vi "Multiple_Windows.vi"() -> ()   [LabVIEW 2013]
uses:
  Global 2.vi
panel:
  in  "Input2":enum32{"Input2"}(tab)
  in  "OK Input 2":bool
  out "Input2_A":dbl
  out "Input2_B":dbl
  out "Input1":enum32{"Input1"}(tab)
  in  "OK Input 1":bool
  out "Input1_A":dbl
  out "Input1_B":dbl
  out "Input1 4":enum32{"Home"}(tab)
  in  "OK Input 3":bool
  in  "close":bool
  in  "Tab Control":enum32{"Home", "Input1", "Input2"}(tab)
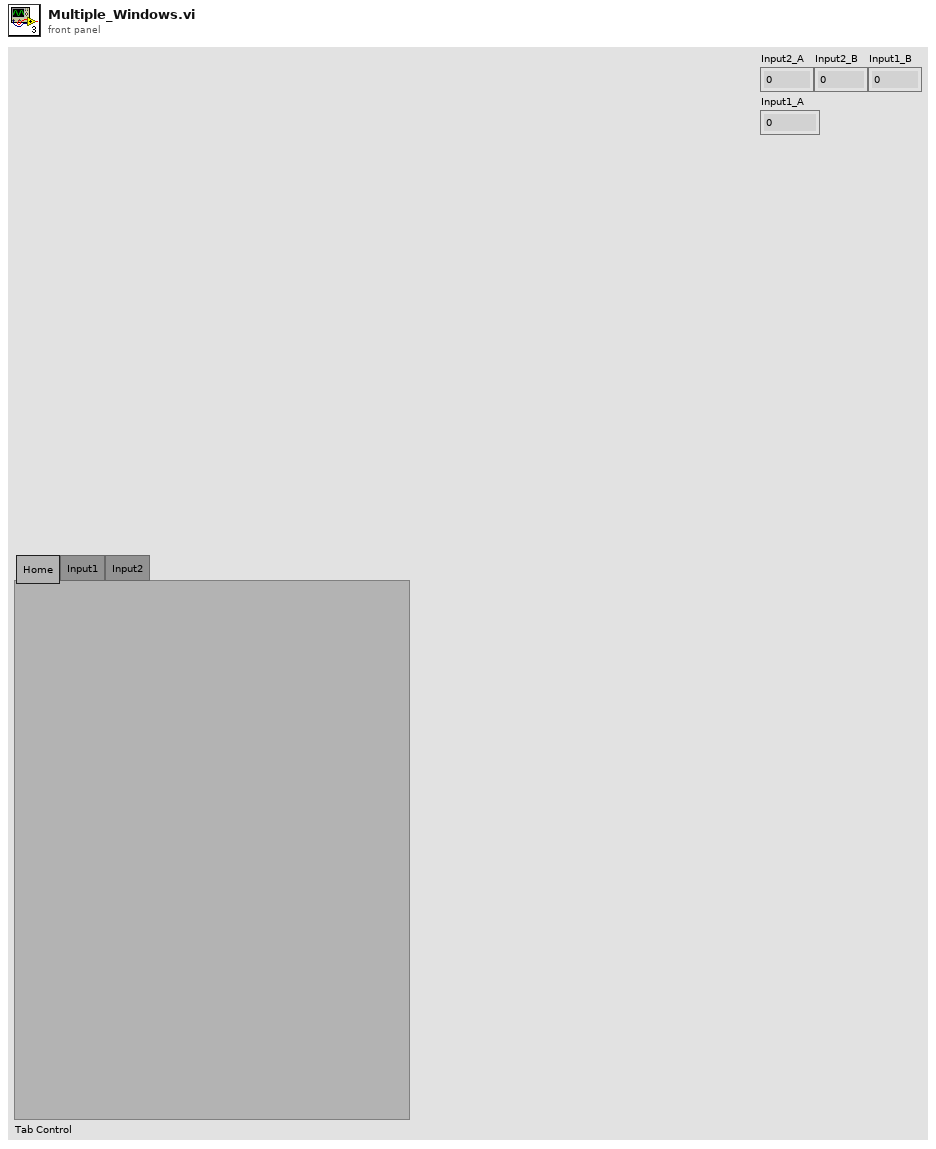
[diagram p1: front panel]
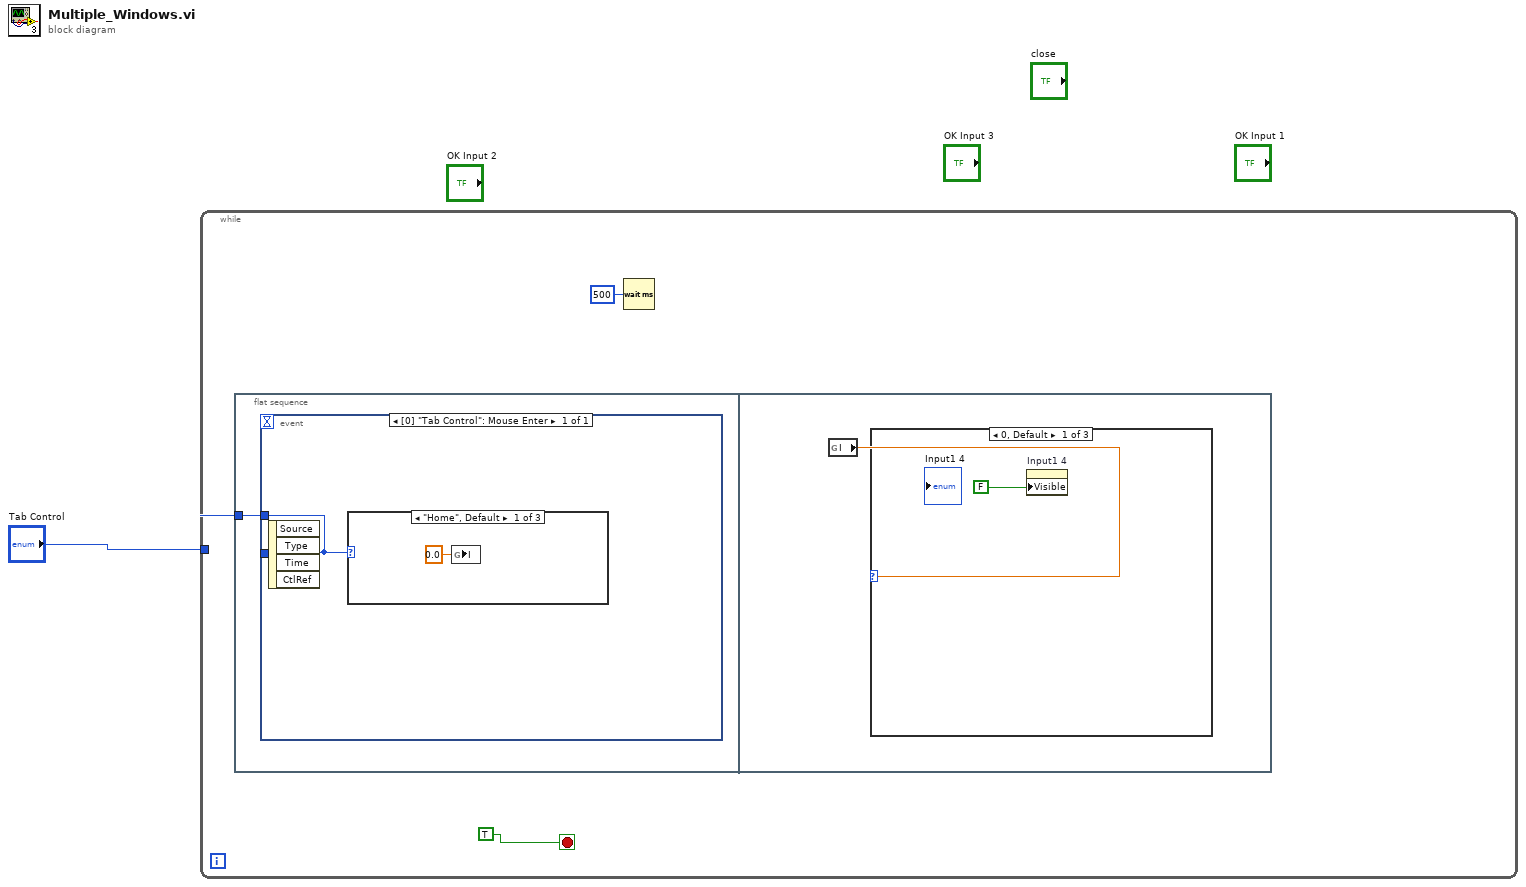
[diagram p0: block diagram]
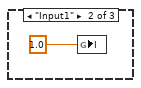
[diagram p2: hidden frame]
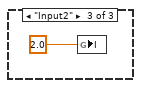
[diagram p3: hidden frame]
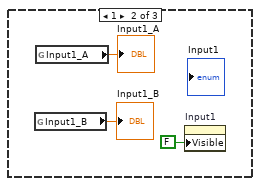
[diagram p4: hidden frame]
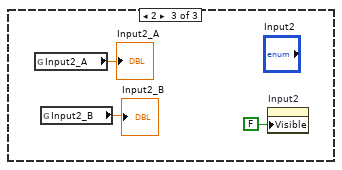
[diagram p5: hidden frame]
diagram:
  n1 = while {
    tunnel: "Tab Control" -> [w3]
    stop <- TRUE stop-if-true
    n2 = flat-sequence {
      tunnel: w3 -> [w5]
      frame #0 {
        n3 = event shown="[0] \"Tab Control\": Mouse Enter" {
          selector: _ -> [_]
          dyn-events: _ -> [_]
          timeout: _ -> [_]
          tunnel: [w6] -> _
          tunnel: w5 -> [w6]
          event "Tab Control": Mouse Enter {
            n4 = event-data() -> ()  [unwired: 1 in, 4 out]
            n5 = case shown="\"Home\", Default" w6 {
              frame "Home", Default {
                n6 = global write "Global 2.vi" "I"(0.0 ("I")) -> ()
              }
              frame "Input1" {
                n7 = global write "Global 2.vi" "I"(1.0 ("Input1_A")) -> ()
              }
              frame "Input2" {
                n8 = global write "Global 2.vi" "I"(2.0 ("Input1_A")) -> ()
              }
            }
          }
        }
      }
      frame #1 {
        n9 = global read "Global 2.vi" "I"() -> (w10:dbl)
        n10 = case shown="0, Default" w10 {
          frame 0, Default {
            n11 = property on="Input1 4" class="TabCtl (strict)"("Visible"=FALSE) -> ()  [unwired: 2 in, 2 out]
          }
          frame 1 {
            n12 = global read "Global 2.vi" "Input1_B"() -> (→"Input1_B":dbl)
            n13 = global read "Global 2.vi" "Input1_A"() -> (→"Input1_A":dbl)
            n14 = property on="Input1" class="TabCtl (strict)"("Visible"=FALSE) -> ()  [unwired: 2 in, 2 out]
          }
          frame 2 {
            n15 = global read "Global 2.vi" "Input2_A"() -> (→"Input2_A":dbl)
            n16 = global read "Global 2.vi" "Input2_B"() -> (→"Input2_B":dbl)
            n17 = property on="Input2" class="TabCtl (strict)"("Visible"=FALSE) -> ()  [unwired: 2 in, 2 out]
          }
        }
      }
    }
    n18 = Wait (ms)(milliseconds to wait=u32 500) -> ()  [unwired: 1 out]
  }
